vi "Destroy DC Power Session.vi"(8 "error in (no error)":errorcluster, 10 "session information":T1, 11 "instrument handle":refnum<k15>) -> (0 "error out":errorcluster)   [LabVIEW 2020, in "NIDCPowerSourceDCVoltage.lvlib"]
doc: "Destroys the given NI DC power instrument handle."
uses:
  NIDCPowerSourceDCVoltage.lvlib
  <vilib>/MeasurementLink/MeasurementLink Session Management Client/RPC Messages/ni_measurementlink_sessionmanagement_v1_SessionInformation.ctl
  <vilib>/MeasurementLink/MeasurementLink Session Management Client/RPC Messages/nidevice_grpc_Session.ctl
  <vilib>/MeasurementLink/MeasurementLink Session Management Client/RPC Messages/ni_measurementlink_sessionmanagement_v1_ChannelMapping.ctl
  <vilib>/MeasurementLink/MeasurementLink Session Management Client/MeasurementLink Session Management Client.lvlib
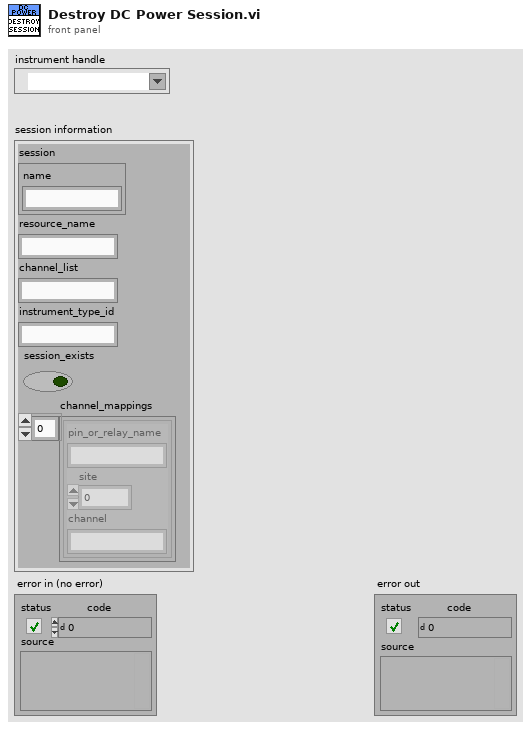
[diagram p1: front panel]
types:
  T1 = typedef "MeasurementLink Session Management Client.lvlib/ni_measurementlink_sessionmanagement_v1_SessionInformation.ctl" = cluster{"session":T2, "resource_name":string, "channel_list":string, "instrument_type_id":string, "session_exists":bool, "channel_mappings":T3[]}
  T2 = typedef "MeasurementLink Session Management Client.lvlib/nidevice_grpc_Session.ctl" = cluster{"name":string}
  T3 = typedef "MeasurementLink Session Management Client.lvlib/ni_measurementlink_sessionmanagement_v1_ChannelMapping.ctl" = cluster{"pin_or_relay_name":string, "site":i32, "channel":string}
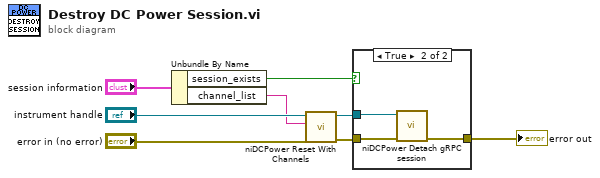
[diagram p0: block diagram]
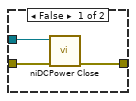
[diagram p2: hidden frame]
diagram:
  n1 = Unbundle By Name("session information") -> ("session_exists"=w5:bool, "channel_list"=w1:string)
  n2 = call <instrlib>:"niDCPower Reset With Channels.vi"("error in (no error)"="error in (no error)", "channel name"=w1, "instrument handle"="instrument handle") -> ("error out"=w7:errorcluster, "instrument handle out"=w6:refnum<k15>)  [unwired: 7 in]
  n3 = case shown="True" w5 {
    tunnel: w6 -> [w11 w12]
    tunnel: w7 -> [w10 w13]
    tunnel: [w9 w14] -> w2
    frame False {
      n4 = call <instrlib>:"niDCPower Close.vi"("error in (no error)"=w10, "instrument handle"=w11) -> ("error out"=w9:errorcluster)  [unwired: 9 out]
    }
    frame True {
      n5 = call <instrlib>:"niDCPower Detach gRPC session.vi"("error in (no error)"=w13, "instrument handle"=w12) -> ("error out"=w14:errorcluster)  [unwired: 9 in]
    }
  }
  "error out" <- w2
